vi "Mixer.Clear Sliders.vi"   [LabVIEW 2020]
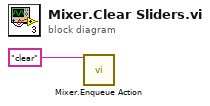
[diagram p0: block diagram]
diagram:
  n1 = call "Mixer.Enqueue Action.vi"("action"="clear") -> ()  [unwired: 14 in, 1 out]
